vi "hold note manage.vi"(7 "keys pressed":T4(array[ring]), 8 "song info":T3, 10 "score info":T2, 11 "hold note key":T1) -> (2 "new score info":T2, 3 "new hold note key":T1)   [LabVIEW 2023]
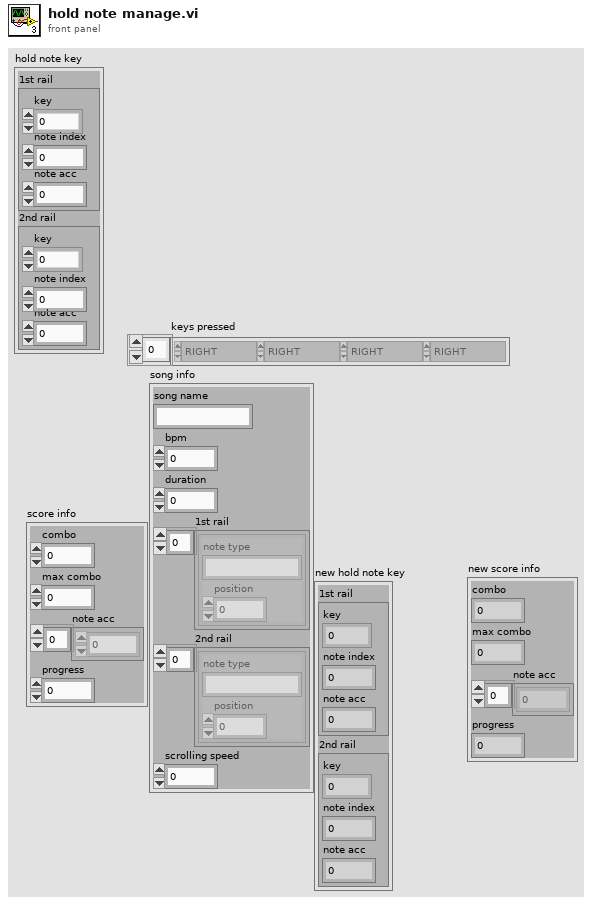
[diagram p1: front panel]
types:
  T1 = cluster{"1st rail":cluster{"key":enum16{"0", "1", "2", "3", "4", "5", "6", "7", "8", "9", "A", "B", "C", "D", "E", "F", "G", "H", "I", "J", "K", "L", "M", "N", "O", "P", "Q", "R", "S", "T", "U", "V", "W", "X", "Y", "Z", "F1", "F2", "F3", "F4", "F5", "F6", "F7", "F8", "F9", "F10", "F11", "F12", "F13", "F14", "F15", "ADD", "BACK", "BACKSLASH", "CAPITAL", "COMMA", "DECIMAL", "DELETE", "DIVIDE", "DOWN", "END", "EQUALS", "ESCAPE", "GRAVE (`)", "HOME", "INSERT", "LBRACKET", "LCONTROL", "LEFT", "L ALT", "LSHIFT", "LWIN", "MINUS", "MULTIPLY", "NEXT", "NUMLOCK", "NUMPAD_0", "NUMPAD_1", "NUMPAD_2", "NUMPAD_3", "NUMPAD_4", "NUMPAD_5", "NUMPAD_6", "NUMPAD_7", "NUMPAD_8", "NUMPAD_9", "PAUSE", "PERIOD", "PRIOR (PG UP)", "RBRACKET", "RCONTROL", "RETURN", "RIGHT", "R ALT", "RSHIFT", "RWIN", "SCROLL", "SEMICOLON", "SLASH", "SPACE", "SUBTRACT", "TAB", "UP", "ENTER (num pad)", "' (quote)"}, "note index":i32, "note acc":i32}, "2nd rail":cluster{"key":enum16{"0", "1", "2", "3", "4", "5", "6", "7", "8", "9", "A", "B", "C", "D", "E", "F", "G", "H", "I", "J", "K", "L", "M", "N", "O", "P", "Q", "R", "S", "T", "U", "V", "W", "X", "Y", "Z", "F1", "F2", "F3", "F4", "F5", "F6", "F7", "F8", "F9", "F10", "F11", "F12", "F13", "F14", "F15", "ADD", "BACK", "BACKSLASH", "CAPITAL", "COMMA", "DECIMAL", "DELETE", "DIVIDE", "DOWN", "END", "EQUALS", "ESCAPE", "GRAVE (`)", "HOME", "INSERT", "LBRACKET", "LCONTROL", "LEFT", "L ALT", "LSHIFT", "LWIN", "MINUS", "MULTIPLY", "NEXT", "NUMLOCK", "NUMPAD_0", "NUMPAD_1", "NUMPAD_2", "NUMPAD_3", "NUMPAD_4", "NUMPAD_5", "NUMPAD_6", "NUMPAD_7", "NUMPAD_8", "NUMPAD_9", "PAUSE", "PERIOD", "PRIOR (PG UP)", "RBRACKET", "RCONTROL", "RETURN", "RIGHT", "R ALT", "RSHIFT", "RWIN", "SCROLL", "SEMICOLON", "SLASH", "SPACE", "SUBTRACT", "TAB", "UP", "ENTER (num pad)", "' (quote)"}, "note index":i32, "note acc":i32}}
  T2 = cluster{"combo":i32, "max combo":i32, "note acc":i32[], "progress":dbl}
  T3 = cluster{"song name":string, "bpm":i32, "duration":i32, "1st rail":cluster{"note type":string, "position":dbl}[], "2nd rail":cluster{"note type":string, "position":dbl}[], "scrolling speed":dbl}
  T4 = enum16{"0", "1", "2", "3", "4", "5", "6", "7", "8", "9", "A", "B", "C", "D", "E", "F", "G", "H", "I", "J", "K", "L", "M", "N", "O", "P", "Q", "R", "S", "T", "U", "V", "W", "X", "Y", "Z", "F1", "F2", "F3", "F4", "F5", "F6", "F7", "F8", "F9", "F10", "F11", "F12", "F13", "F14", "F15", "ADD", "BACK", "BACKSLASH", "CAPITAL", "COMMA", "DECIMAL", "DELETE", "DIVIDE", "DOWN", "END", "EQUALS", "ESCAPE", "GRAVE (`)", "HOME", "INSERT", "LBRACKET", "LCONTROL", "LEFT", "L ALT", "LSHIFT", "LWIN", "MINUS", "MULTIPLY", "NEXT", "NUMLOCK", "NUMPAD_0", "NUMPAD_1", "NUMPAD_2", "NUMPAD_3", "NUMPAD_4", "NUMPAD_5", "NUMPAD_6", "NUMPAD_7", "NUMPAD_8", "NUMPAD_9", "PAUSE", "PERIOD", "PRIOR (PG UP)", "RBRACKET", "RCONTROL", "RETURN", "RIGHT", "R ALT", "RSHIFT", "RWIN", "SCROLL", "SEMICOLON", "SLASH", "SPACE", "SUBTRACT", "TAB", "UP", "ENTER (num pad)", "' (quote)"}[]
  T5 = enum16{"0", "1", "2", "3", "4", "5", "6", "7", "8", "9", "A", "B", "C", "D", "E", "F", "G", "H", "I", "J", "K", "L", "M", "N", "O", "P", "Q", "R", "S", "T", "U", "V", "W", "X", "Y", "Z", "F1", "F2", "F3", "F4", "F5", "F6", "F7", "F8", "F9", "F10", "F11", "F12", "F13", "F14", "F15", "ADD", "BACK", "BACKSLASH", "CAPITAL", "COMMA", "DECIMAL", "DELETE", "DIVIDE", "DOWN", "END", "EQUALS", "ESCAPE", "GRAVE (`)", "HOME", "INSERT", "LBRACKET", "LCONTROL", "LEFT", "L ALT", "LSHIFT", "LWIN", "MINUS", "MULTIPLY", "NEXT", "NUMLOCK", "NUMPAD_0", "NUMPAD_1", "NUMPAD_2", "NUMPAD_3", "NUMPAD_4", "NUMPAD_5", "NUMPAD_6", "NUMPAD_7", "NUMPAD_8", "NUMPAD_9", "PAUSE", "PERIOD", "PRIOR (PG UP)", "RBRACKET", "RCONTROL", "RETURN", "RIGHT", "R ALT", "RSHIFT", "RWIN", "SCROLL", "SEMICOLON", "SLASH", "SPACE", "SUBTRACT", "TAB", "UP", "ENTER (num pad)", "' (quote)"}
  T6 = cluster{"y":enum16{"0", "1", "2", "3", "4", "5", "6", "7", "8", "9", "A", "B", "C", "D", "E", "F", "G", "H", "I", "J", "K", "L", "M", "N", "O", "P", "Q", "R", "S", "T", "U", "V", "W", "X", "Y", "Z", "F1", "F2", "F3", "F4", "F5", "F6", "F7", "F8", "F9", "F10", "F11", "F12", "F13", "F14", "F15", "ADD", "BACK", "BACKSLASH", "CAPITAL", "COMMA", "DECIMAL", "DELETE", "DIVIDE", "DOWN", "END", "EQUALS", "ESCAPE", "GRAVE (`)", "HOME", "INSERT", "LBRACKET", "LCONTROL", "LEFT", "L ALT", "LSHIFT", "LWIN", "MINUS", "MULTIPLY", "NEXT", "NUMLOCK", "NUMPAD_0", "NUMPAD_1", "NUMPAD_2", "NUMPAD_3", "NUMPAD_4", "NUMPAD_5", "NUMPAD_6", "NUMPAD_7", "NUMPAD_8", "NUMPAD_9", "PAUSE", "PERIOD", "PRIOR (PG UP)", "RBRACKET", "RCONTROL", "RETURN", "RIGHT", "R ALT", "RSHIFT", "RWIN", "SCROLL", "SEMICOLON", "SLASH", "SPACE", "SUBTRACT", "TAB", "UP", "ENTER (num pad)", "' (quote)"}, i32, i32}
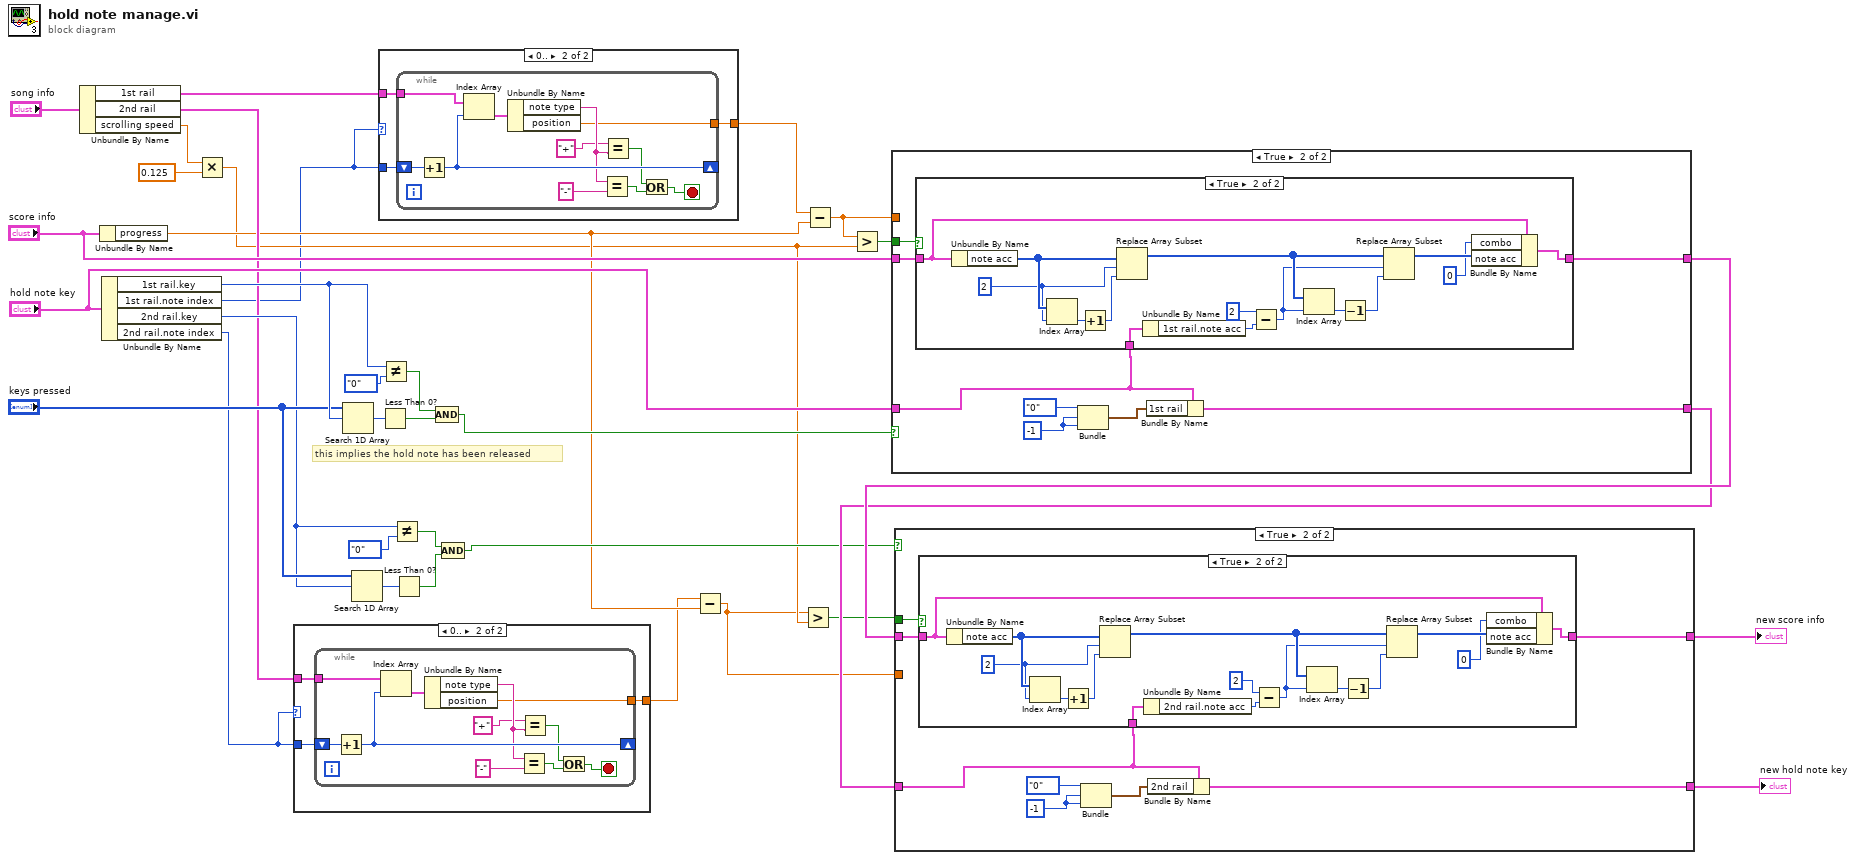
[diagram p0: block diagram]
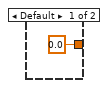
[diagram p2: hidden frame]
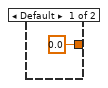
[diagram p3: hidden frame]
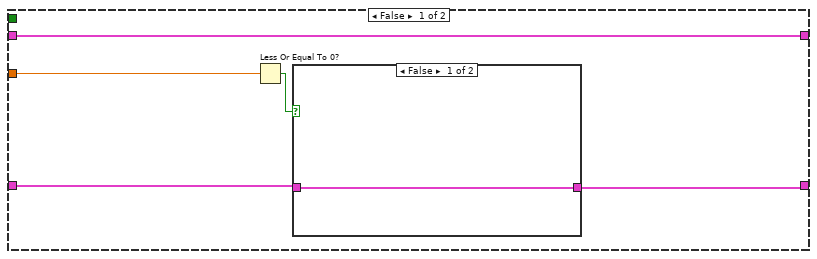
[diagram p4: hidden frame]
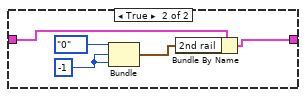
[diagram p5: hidden frame]
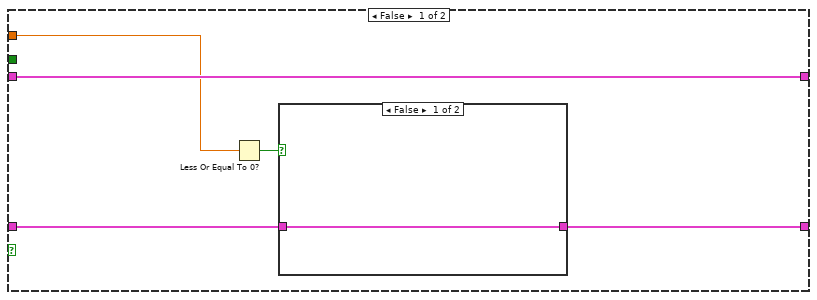
[diagram p7: hidden frame]
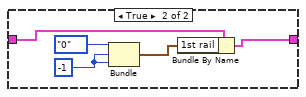
[diagram p8: hidden frame]
diagram:
  # "this implies the hold note has been released"
  n1 = Unbundle By Name("song info") -> ("1st rail"=w28:cluster{"note type":string, "position":dbl}[], "2nd rail"=w11:cluster{"note type":string, "position":dbl}[], "scrolling speed"=w26:dbl)
  n2 = Unbundle By Name("score info") -> ("progress"=w10:dbl)
  n3 = Unbundle By Name("hold note key") -> ("1st rail.key"=w32:T5, "1st rail.note index"=w4:i32, "2nd rail.key"=w15:T5, "2nd rail.note index"=w3:i32)
  n4 = Multiply(x=w26, y=0.125) -> (x*y=w8:dbl)
  n5 = case shown="0.." w3 {
    tunnel: w11 -> [_ w38]
    tunnel: w3 -> [_ w37]
    tunnel: [0.0 ("position") w36] -> w9
    frame Default {
    }
    frame 0.. {
      n6 = while {
        tunnel: w38 -> [w48]
        shift-right: [w47] -> _
        shift-left: w37 -> [w49]
        tunnel: [w39] -> w36
        stop <- w40 stop-if-true
        n7 = Increment(x=w49) -> (x+1=w47:i32)
        n8 = Index Array(array=w48, index=w47) -> (element=w46:cluster{"note type":string, "position":dbl})
        n9 = Unbundle By Name(w46) -> ("note type"=w44:string, "position"=w39:dbl)
        n10 = Equal?(x=w44, y="-") -> (x = y?=w42:bool)
        n11 = Equal?(x="+" ("y"), y=w44) -> (x = y?=w41:bool)
        n12 = Or(x=w41, y=w42) -> (x .or. y?=w40:bool)
      }
    }
  }
  n13 = Search 1D Array(1D array="keys pressed", element=w32) -> (index of element=w34:i32)  [unwired: 1 in]
  n14 = Search 1D Array(1D array="keys pressed", element=w15) -> (index of element=w14:i32)  [unwired: 1 in]
  n15 = case shown="0.." w4 {
    tunnel: w4 -> [_ w53]
    tunnel: w28 -> [_ w52]
    tunnel: [0.0 ("position") w51] -> w27
    frame Default {
    }
    frame 0.. {
      n16 = while {
        tunnel: w52 -> [w63]
        shift-right: [w62] -> _
        shift-left: w53 -> [w64]
        tunnel: [w54] -> w51
        stop <- w55 stop-if-true
        n17 = Increment(x=w64) -> (x+1=w62:i32)
        n18 = Index Array(array=w63, index=w62) -> (element=w61:cluster{"note type":string, "position":dbl})
        n19 = Unbundle By Name(w61) -> ("note type"=w59:string, "position"=w54:dbl)
        n20 = Equal?(x=w59, y="-") -> (x = y?=w57:bool)
        n21 = Equal?(x="+" ("y"), y=w59) -> (x = y?=w56:bool)
        n22 = Or(x=w56, y=w57) -> (x .or. y?=w55:bool)
      }
    }
  }
  n23 = Less Than 0?(x=w34) -> (x < 0?=w33:bool)
  n24 = Not Equal?(x=w32, y=T5."0") -> (x != y?=w30:bool)
  n25 = Not Equal?(x=w15, y=T5."0") -> (x != y?=w18:bool)
  n26 = Less Than 0?(x=w14) -> (x < 0?=w13:bool)
  n27 = Compound Arithmetic op=AND(w30, w33) -> (w24:bool)
  n28 = Compound Arithmetic op=AND(w18, w13) -> (w12:bool)
  n29 = Subtract(x=w9, y=w10) -> (x-y=w1:dbl)
  n30 = Greater?(x=w1, y=w8) -> (0:w7:bool)
  n31 = Subtract(x=w27, y=w10) -> (x-y=w2:dbl)
  n32 = Greater?(x=w2, y=w8) -> (0:w23:bool)
  n33 = case shown="True" w24 {
    tunnel: w23 -> [_ w83]
    tunnel: "score info" -> [w69 w82]
    tunnel: "hold note key" -> [w66 w76]
    tunnel: [w65 w80] -> w19
    tunnel: [w69 w77] -> w20
    tunnel: w2 -> [w67 _]
    frame False {
      n34 = Less Or Equal To 0?(x=w67) -> (x <= 0?=w68:bool)
      n35 = case shown="False" w68 {
        tunnel: w66 -> [w70 w72]
        tunnel: [w70 w71] -> w65
        frame False {
        }
        frame True {
          w73 = -1
          n36 = Bundle("y"=T5."0", w73, w73) -> (w74:T6)  [unwired: 1 in]
          n37 = Bundle By Name(cluster=w72, "1st rail"=w74) -> (w71:T1)
        }
      }
    }
    frame True {
      w78 = -1
      n38 = case shown="True" w83 {
        tunnel: w82 -> [w84 w99]
        tunnel: [w84 w94] -> w77
        tunnel: w76 -> [_ w93]
        frame False {
        }
        frame True {
          w95 = 2 ("index")
          n39 = Unbundle By Name(w99) -> ("note acc"=w97:i32[])
          n40 = Index Array(array=w97, index=w95) -> (element=w98:i32)
          n41 = Increment(x=w98) -> (x+1=w96:i32)
          n42 = Replace Array Subset(array=w97, new element=w96, index=w95) -> (w90:i32[])
          n43 = Unbundle By Name(w93) -> ("1st rail.note acc"=w92:i32)
          n44 = Subtract(x=2, y=w92) -> (x-y=w89:i32)
          n45 = Index Array(array=w90, index=w89) -> (element=w88:i32)
          n46 = Decrement(x=w88) -> (x-1=w87:i32)
          n47 = Replace Array Subset(array=w90, new element=w87, index=w89) -> (w86:i32[])
          n48 = Bundle By Name(cluster=w99, "combo"=0, "note acc"=w86) -> (w94:T2)
        }
      }
      n49 = Bundle("y"=T5."0", w78, w78) -> (w79:T6)  [unwired: 1 in]
      n50 = Bundle By Name(cluster=w76, "1st rail"=w79) -> (w80:T1)
    }
  }
  n51 = case shown="True" w12 {
    tunnel: w7 -> [_ w118]
    tunnel: w20 -> [w104 w117]
    tunnel: w19 -> [w102 w111]
    tunnel: [w101 w115] -> w5
    tunnel: [w104 w112] -> w6
    tunnel: w1 -> [w100 _]
    frame False {
      n52 = Less Or Equal To 0?(x=w100) -> (x <= 0?=w103:bool)
      n53 = case shown="False" w103 {
        tunnel: w102 -> [w105 w107]
        tunnel: [w105 w106] -> w101
        frame False {
        }
        frame True {
          w108 = -1
          n54 = Bundle("y"=T5."0", w108, w108) -> (w109:T6)  [unwired: 1 in]
          n55 = Bundle By Name(cluster=w107, "2nd rail"=w109) -> (w106:T1)
        }
      }
    }
    frame True {
      w113 = -1
      n56 = case shown="True" w118 {
        tunnel: w117 -> [w119 w134]
        tunnel: [w119 w129] -> w112
        tunnel: w111 -> [_ w128]
        frame False {
        }
        frame True {
          w130 = 2 ("index")
          n57 = Unbundle By Name(w134) -> ("note acc"=w132:i32[])
          n58 = Index Array(array=w132, index=w130) -> (element=w133:i32)
          n59 = Increment(x=w133) -> (x+1=w131:i32)
          n60 = Replace Array Subset(array=w132, new element=w131, index=w130) -> (w125:i32[])
          n61 = Unbundle By Name(w128) -> ("2nd rail.note acc"=w127:i32)
          n62 = Subtract(x=2, y=w127) -> (x-y=w124:i32)
          n63 = Index Array(array=w125, index=w124) -> (element=w123:i32)
          n64 = Decrement(x=w123) -> (x-1=w122:i32)
          n65 = Replace Array Subset(array=w125, new element=w122, index=w124) -> (w121:i32[])
          n66 = Bundle By Name(cluster=w134, "combo"=0, "note acc"=w121) -> (w129:T2)
        }
      }
      n67 = Bundle("y"=T5."0", w113, w113) -> (w114:T6)  [unwired: 1 in]
      n68 = Bundle By Name(cluster=w111, "2nd rail"=w114) -> (w115:T1)
    }
  }
  "new score info" <- w6
  "new hold note key" <- w5
